vi "build.vi"(8 "error in (no error)":errorcluster, 10 "Instance in":refnum<class "IInstance.lvclass">, 11 "IInstanceBuilder in":refnum<class "IInstanceBuilder.lvclass">) -> (0 "error out":errorcluster, 2 "Instance out":refnum<class "IInstance.lvclass">, 3 "IInstanceBuilder out":refnum<class "IInstanceBuilder.lvclass">)   [LabVIEW 2022 SP3, in "openDAQ.lvlib" / "IBaseObject.lvlib" / "IInstanceBuilder.lvlib" / "IInstanceBuilder.lvclass"]
uses:
  <instrlib>/openDAQ/Public/Classes/IInstanceBuilder/IInstanceBuilder.lvclass
  C:/Program Files (x86)/National Instruments/LabVIEW 2022/instr.lib/openDAQ/Public/Classes/IBaseObject/IBaseObject.lvclass
  <instrlib>/openDAQ/Public/Classes/IInstance/IInstance.lvclass
  <instrlib>/openDAQ/Public/Classes/IBaseObject/IBaseObject.lvclass/IBaseObject.ctl
  <instrlib>/openDAQ/Public/Classes/IBaseObject/Accessor/Read reference.vi
  <instrlib>/openDAQ/Public/Classes/IBaseObject/Accessor/Write reference.vi
  <instrlib>/openDAQ/Binaries/Windows/x86/copendaq32.dll
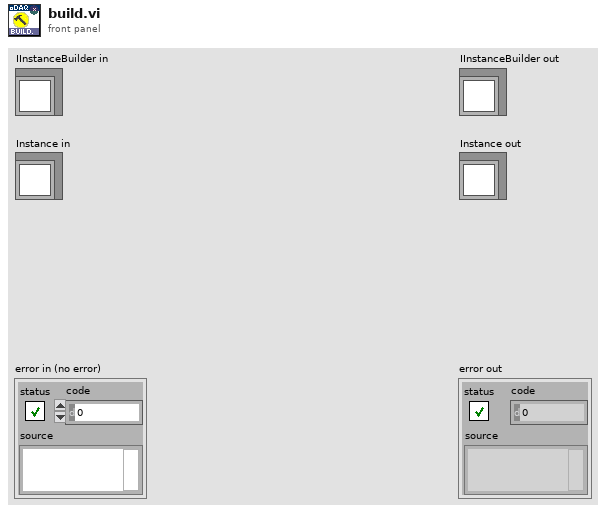
[diagram p1: front panel]
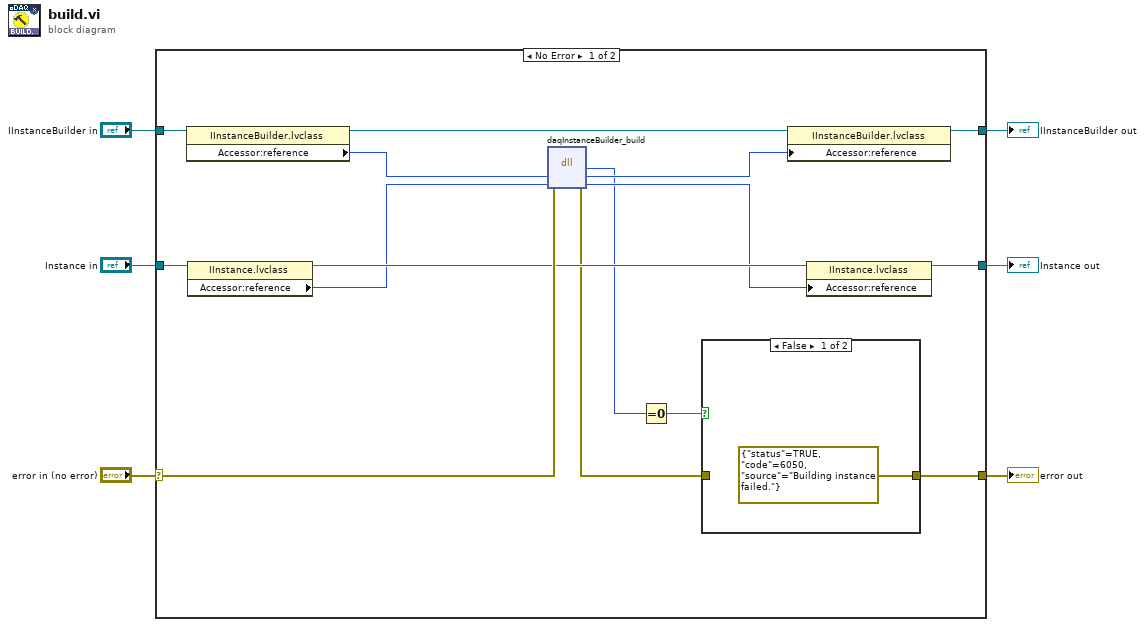
[diagram p0: block diagram]
diagram:
  n1 = case shown="No Error" "error in (no error)" {
    selector: "error in (no error)" -> [w21 w26]
    tunnel: [w8 w26] -> w3
    tunnel: [w18 w25] -> w5
    tunnel: "IInstanceBuilder in" -> [w20 w25]
    tunnel: "Instance in" -> [w15 w24]
    tunnel: [w13 w24] -> w2
    frame No Error {
      n2 = property class="IInstanceBuilder.lvclass"(reference=w20) -> (reference out=w19:refnum<class "IInstanceBuilder.lvclass">, "Accessor:reference"=w17:i64)  [unwired: 1 in, 1 out]
      n3 = property class="IInstance.lvclass"(reference=w15) -> (reference out=w14:refnum<class "IInstance.lvclass">, "Accessor:reference"=w12:i64)  [unwired: 1 in, 1 out]
      n4 = dll-call lib="C:/Program Files (x86)/National Instruments/LabVIEW 2022/instr.lib/openDAQ/Binaries/Windows/x86/copendaq*.*" fn="daqInstanceBuilder_build"(error in=w21, "instanceBuilder"=w17, "instance"=w12) -> (error out=w7:errorcluster, "return type"=w10:u32, "instanceBuilder"=w16:i64, "instance"=w11:i64)  [unwired: 2 in, 1 out]
      n5 = Equal To 0?(x=w10) -> (x = 0?=w9:bool)
      n6 = case shown="False" w9 {
        tunnel: [errorcluster {"status"=TRUE, "code"=6050, "source"="Building instance failed."} ("error out") w23] -> w8
        tunnel: w7 -> [_ w23]
        frame False {
        }
        frame True {
        }
      }
      n7 = property class="IInstanceBuilder.lvclass"(reference=w19, "Accessor:reference"=w16) -> (reference out=w18:refnum<class "IInstanceBuilder.lvclass">)  [unwired: 1 in, 1 out]
      n8 = property class="IInstance.lvclass"(reference=w14, "Accessor:reference"=w11) -> (reference out=w13:refnum<class "IInstance.lvclass">)  [unwired: 1 in, 1 out]
    }
    frame Error {
    }
  }
  "error out" <- w3
  "IInstanceBuilder out" <- w5
  "Instance out" <- w2
